vi "Begin.vi"(11 "Image Size":T1=enum."160x120") -> (0 "error out":errorcluster)   [LabVIEW 2013]
doc: "Called before other user functions, this VI is expected to open initial I/O refnums, load in file data, and do all program initialization. Notice that the <B>error out</B> terminal is simply used for data flow. Wiring it to other structures or subVIs ensures that this VI runs first."
uses:
  <vilib>/Rock Robotics/WPI/Camera/WPI_CameraImageSize.ctl
  <vilib>/Rock Robotics/WPI/Camera/WPI_CameraWhite Balance Values.ctl
  <vilib>/Rock Robotics/WPI/Camera/WPI_CameraExposure Values.ctl
  <vilib>/Rock Robotics/WPI/Camera/WPI_CameraFrameRate.ctl
  <vilib>/Rock Robotics/WPI/SafetyOutput/WPI_SafetyOutputConfigMenu.ctl
  <vilib>/Rock Robotics/WPI/DriverStation/WPI_DriverStationRobotMode2.ctl
  <vilib>/Rock Robotics/WPI/Joystick/WPI_JoystickDeviceEnum.ctl
  <vilib>/Rock Robotics/WPI/CAN/Jaguar/SubVIs/WPI_CANJaguar_ControlMode.ctl
  <vilib>/Rock Robotics/SystemInterfaces/DIO/FPGA_DIOPWMChannel.ctl
  <vilib>/Rock Robotics/SystemInterfaces/Typedef/FPGA_TypedefDigitalModule.ctl
  <vilib>/Rock Robotics/SystemInterfaces/DIO/FPGA_DIOChannel.ctl
  <vilib>/Rock Robotics/SystemInterfaces/AI/FPGA_AIChannel.ctl
  Robot Global Data.vi
  <vilib>/Rock Robotics/WPI/RobotDrive/WPI_RobotDriveOpen4MotorWithCANJaguar.vi
  <vilib>/Rock Robotics/WPI/MotorControl/WPI_MotorControlOpenCANJaguar.vi
  <vilib>/Rock Robotics/WPI/MotorControl/WPI_MotorControlOpen Victor.vi
  <vilib>/Rock Robotics/WPI/Relay/WPI_RelayDirection.ctl
  <vilib>/Rock Robotics/SystemInterfaces/DIO/FPGA_DIORelayChannel.ctl
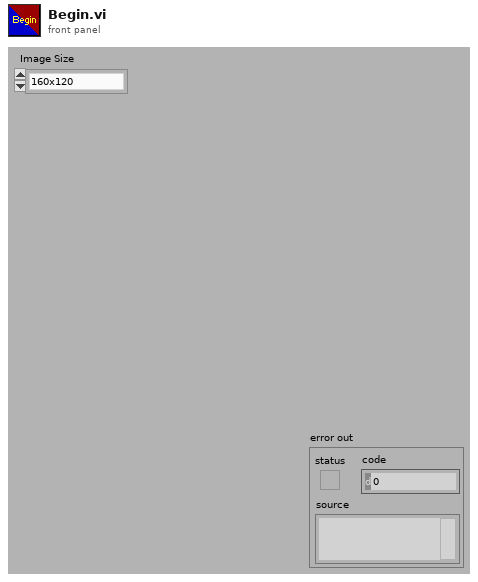
[diagram p1: front panel]
types:
  T1 = typedef "WPI_CameraImageSize.ctl" = enum16{"640x480", "320x240", "160x120"}
  T2 = typedef "FPGA_AIChannel.ctl" = enum8{"AI 1", "AI 2", "AI 3", "AI 4", "AI 5", "AI 6", "AI 7", "AI 8", "Invalid"}
  T3 = typedef "FPGA_DIOChannel.ctl" = enum8{"DIO 1", "DIO 2", "DIO 3", "DIO 4", "DIO 5", "DIO 6", "DIO 7", "DIO 8", "DIO 9", "DIO 10", "DIO 11", "DIO 12", "DIO 13", "DIO 14", "Invalid"}
  T4 = typedef "FPGA_DIOPWMChannel.ctl" = enum8{"PWM 1", "PWM 2", "PWM 3", "PWM 4", "PWM 5", "PWM 6", "PWM 7", "PWM 8", "PWM 9", "PWM 10", "Invalid"}
  T5 = typedef "FPGA_TypedefDigitalModule.ctl" = enum16{"Digital Module 1", "Digital Module 2"}
  T6 = typedef "WPI_CANJaguar_ControlMode.ctl" = enum8{"Percent VBus", "Current", "Speed", "Position", "Voltage"}
  T7 = typedef "WPI_JoystickDeviceEnum.ctl" = enum16{"USB 1", "USB 2", "USB 3", "USB 4", "Kinect 1", "Kinect 2"}
  T8 = typedef "WPI_DriverStationRobotMode2.ctl" = enum16{"Autonomous Disabled", "Autonomous Enabled", "Teleop Disabled", "Teleop Enabled", "Timeout", "Finish", "Test Disabled", "Test Enabled"}
  T9 = typedef "WPI_SafetyOutputConfigMenu.ctl" = enum16{"Enable", "Disable"}
  T10 = typedef "WPI_CameraFrameRate.ctl" = u32
  T11 = typedef "WPI_CameraExposure Values.ctl" = enum16{"Auto", "Flicker-free 50 Hz", "Flicker-free 60 Hz", "Hold current"}
  T12 = typedef "WPI_CameraWhite Balance Values.ctl" = enum16{"Auto", "Fixed indoor", "Fixed outdoor 1", "Fixed outdoor 2", "Fixed fluorescent 1", "Fixed fluorescent 2", "Hold current"}
  T13 = typedef "WPI_RelayDirection.ctl" = enum16{"Both directions", "Forward only", "Reverse only"}
  T14 = typedef "FPGA_DIORelayChannel.ctl" = enum8{"Relay 1", "Relay 2", "Relay 3", "Relay 4", "Relay 5", "Relay 6", "Relay 7", "Relay 8", "Invalid"}
  T15 = typedef "WPI_RelayDevRef.ctl" = cluster{"DevStatus":errorcluster, "Relay Channel":T14, "Digital Module":T5, "Relay Direction":T13}
  T16 = typedef "WPI_CameraDevRef.ctl" = cluster{"Camera Address":string, "CameraStatus":errorcluster, "Acquire Image Notifier":refnum<notifier>}
  T17 = typedef "WPI_RobotDriveDevRef.ctl" = cluster{"DevStatus":errorcluster, "Motors[]":T18[], "Square Inputs":bool, "Max Output":dbl, "Isochronous":bool}
  T18 = typedef "WPI_MotorControlDeviceRef.ctl" = cluster{"DeviceStatus":errorcluster, "Type":enum16{"PWM", "CAN"}, "PWM":cluster{"Digital Module":T5, "PWM Channel":T4, "DeadBand":T19}, "CAN":cluster{"Device Number":u8, "Control Mode":T6, "Semaphore":T20, "Max Vout":dbl}, "Invert":bool, "TransformRef":T21, "InvTransformRef":T21}
  T19 = typedef "WPI_PWMDeadband.ctl" = cluster{"Name":string, "maxPositivePwm":i32, "minPositivePwm":i32, "centerPwm":i32, "maxNegativePwm":i32, "minNegativePwm":i32, "angularRange":u16}
  T20 = typedef "Semaphore RefNum" = refnum<k1>
  T21 = typedef "WPI_PWMTransform_ConPane.ctl" = refnum<vi>
  T22 = typedef "WPI_ServoDeviceRef.ctl" = cluster{"DeviceStatus":errorcluster, "Digital Module":T5, "PWM Channel":T4, "DeadBand":T19}
  T23 = typedef "WPI_JoystickDevRef.ctl" = cluster{"Device":T7}
  T24 = typedef "WPI_AnalogChannelDevRef.ctl" = cluster{"DevStatus":errorcluster, "Analog Module":T25, "Analog Channel":T2}
  T25 = typedef "FPGA_TypedefAnalogModule.ctl" = enum16{"Analog Module 1", "Analog Module 2"}
  T26 = typedef "WPI_DigitalInputDevRef.ctl" = cluster{"DevStatus":errorcluster, "DIO Channel":T3, "Digital Module":T5}
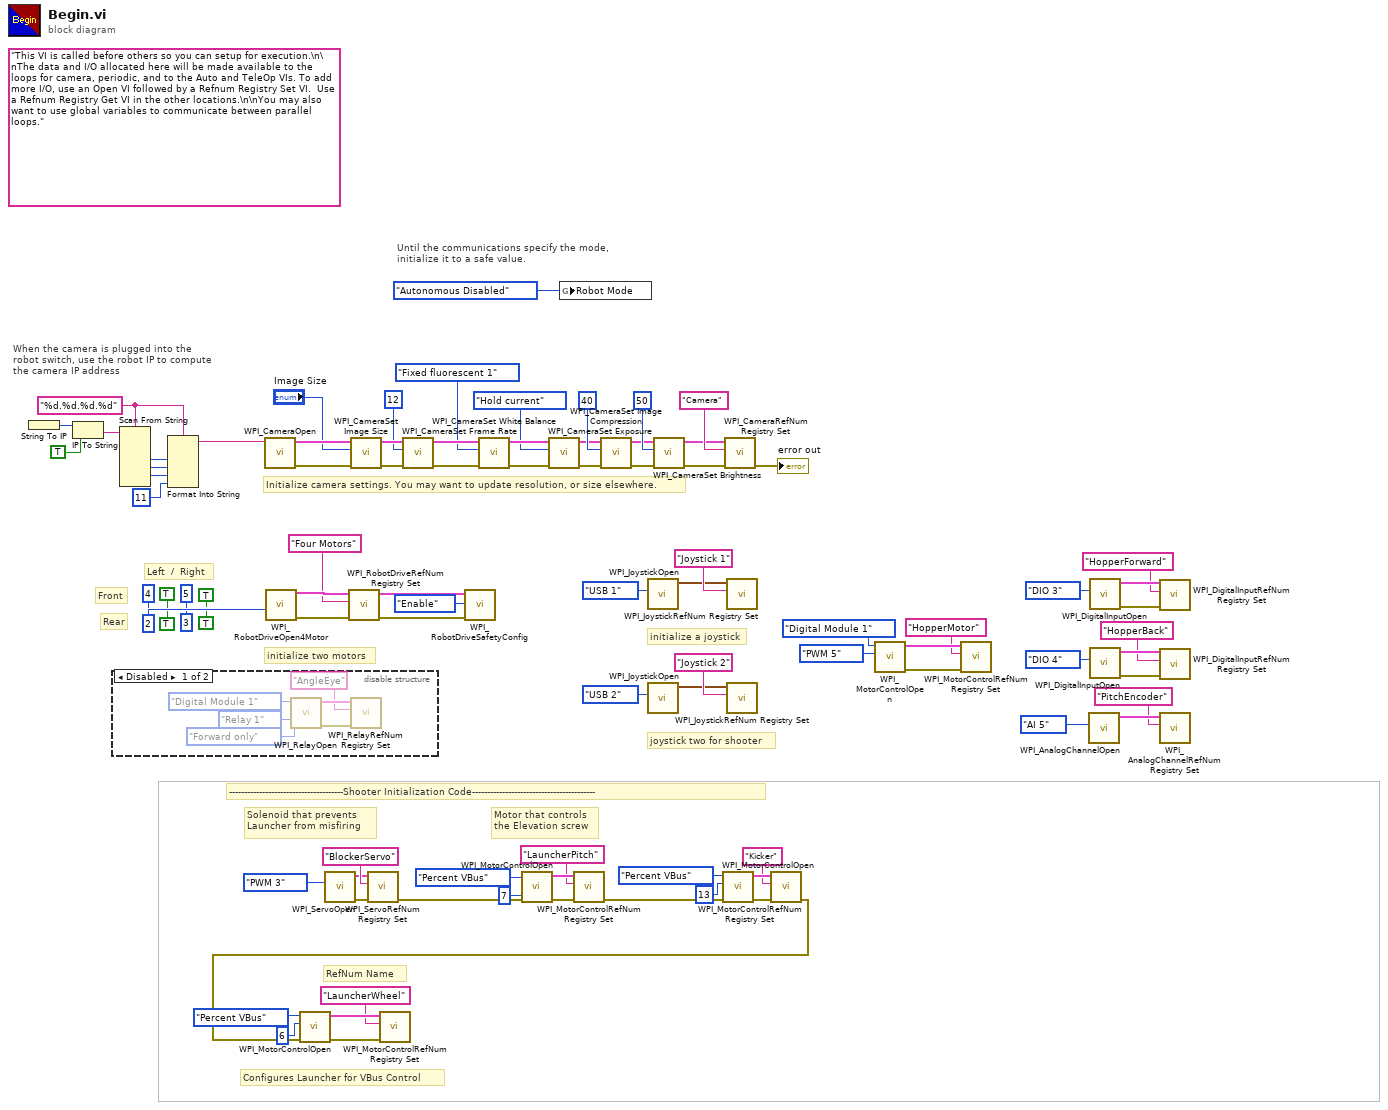
[diagram p0: block diagram]
diagram:
  w59 = "%d.%d.%d.%d" ("format string")
  (unwired) "This VI is called before others so you can setup for execution.\n\nThe data and I/O allocated here will be made available to the loops for camera, periodic, and to the Auto and TeleOp VIs. To add more I/O, use an Open VI followed by a Refnum Registry Set VI.  Use a Refnum Registry Get VI in the other locations.\n\nYou may also want to use global variables to communicate between parallel loops."
  # "Configures Launcher for VBus Control"
  # "RefNum Name"
  # "Motor that controls\nthe Elevation screw"
  # "Solenoid that prevents\nLauncher from misfiring"
  # "--------------------------------------Shooter Initialization Code-----------------------------------------"
  # "joystick two for shooter"
  # "Left  /  Right"
  # "Rear"
  # "Front"
  # "initialize a joystick"
  # "Until the communications specify the mode,\ninitialize it to a safe value."
  # "When the camera is plugged into the\nrobot switch, use the robot IP to compute\nthe camera IP address"
  # "initialize two motors"
  # "Initialize camera settings. You may want to update resolution, or size elsewhere."
  n1 = String To IP() -> (0:w66:u32)  [unwired: 1 in]
  n2 = IP To String(1:TRUE ("dot notation? (F)"), 2:w66) -> (0:w64:string)
  n3 = disable-structure shown="Disabled" {
    frame Disabled {
      n4 = call <vilib>:"WPI_RelayOpen.vi"("Relay Direction"=WPI_RelayDirection."Forward only", "Relay Channel"=FPGA_DIORelayChannel."Relay 1", "Digital Module (Module 1)"=FPGA_TypedefDigitalModule."Digital Module 1") -> ("error out"=w95:errorcluster, "RelayDevRef"=w96:T15)  [unwired: 7 in]
      n5 = call <vilib>:"WPI_RelayRefNum Registry Set.vi"("error in (no error)"=w95, "refnum name"="AngleEye", "RelayDevRef"=w96) -> ()  [unwired: 7 in, 2 out]
    }
    frame Enabled {
    }
  }
  n6 = Scan From String(format string=w59, input string=w64) -> (output 1=w63:i32, output 2=w62:i32, output 3=w61:i32)  [unwired: 7 in, 3 out]
  n7 = Format Into String(format string=w59, w63, w62, w61, 11 ("Compression")) -> (resulting string=w55:string)  [unwired: 2 in, 1 out]
  n8 = call <vilib>:"WPI_CameraOpen.vi"("Camera Address"=w55) -> ("error out"=w78:errorcluster, "CameraDevRef"=w79:T16)  [unwired: 1 in, 8 out]
  n9 = call-poly <vilib>:"WPI_RobotDriveOpen4Motor.vi"("Rear Left Motor"=u8 2, "Rear Left Motor Inverted"=TRUE, "Rear Right Motor Inverted"=TRUE, "Rear Right Motor"=u8 3, "Front Left Motor"=u8 4, "Front Right Motor"=u8 5, "Front Left Motor Inverted"=TRUE, "Front Right Motor Inverted"=TRUE) -> ("RobotDriveDevRef"=w89:T17, "error out"=w87:errorcluster)  [unwired: 6 in]
  n10 = call <vilib>:"WPI_ServoOpen.vi"("PWM Channel"=FPGA_DIOPWMChannel."PWM 3") -> ("error out"=w40:errorcluster, "ServoDeviceRef"=w19:T22)  [unwired: 9 in]
  n11 = call <vilib>:"WPI_RobotDriveRefNum Registry Set.vi"("error in (no error)"=w87, "refnum name"="Four Motors", "RobotDriveDevRef"=w89) -> ("error out"=w20:errorcluster, "RobotDriveDevRef"=w58:T17)  [unwired: 7 out]
  n12 = call <vilib>:"WPI_CameraSet Image Size.vi"("error in (no error)"=w78, "Image Size"="Image Size", "CameraDevRef"=w79) -> ("error out"=w77:errorcluster, "CameraDevRef Out"=w80:T16)  [unwired: 7 out]
  n13 = call <vilib>:"WPI_ServoRefNum Registry Set.vi"("error in (no error)"=w40, "refnum name"="BlockerServo", "ServoDeviceRef"=w19) -> ("error out"=w23:errorcluster)  [unwired: 7 in, 1 out]
  n14 = call <vilib>:"WPI_CameraSet Frame Rate.vi"("error in (no error)"=w77, "Frame Rate (fps)"=T10 12, "CameraDevRef"=w80) -> ("error out"=w76:errorcluster, "CameraDevRef Out"=w82:T16)  [unwired: 7 out]
  n15 = call <vilib>:"WPI_RobotDriveSafetyConfig.vi"("error in (no error)"=w20, "mode"=WPI_SafetyOutputConfigMenu."Enable", "RobotDriveDevRef"=w58) -> ()  [unwired: 7 in, 2 out]
  n16 = call <vilib>:"WPI_CameraSet White Balance.vi"("error in (no error)"=w76, "White Balance"=WPI_CameraWhite_Balance_Values."Fixed fluorescent 1", "CameraDevRef"=w82) -> ("error out"=w75:errorcluster, "CameraDevRef Out"=w81:T16)  [unwired: 7 out]
  n17 = call-poly <vilib>:"WPI_MotorControlOpen.vi"("error in (no error)"=w23, "Device Number"=u8 7, "Control Mode"=WPI_CANJaguar_ControlMode."Percent VBus") -> ("error out"=w35:errorcluster, "MotorControlDeviceRef"=w36:T18)  [unwired: 7 in]
  n18 = call <vilib>:"WPI_CameraSet Exposure.vi"("error in (no error)"=w75, "Exposure"=WPI_CameraExposure_Values."Hold current", "CameraDevRef"=w81) -> ("error out"=w74:errorcluster, "CameraDevRef Out"=w84:T16)  [unwired: 7 out]
  n19 = global write "Robot Global Data.vi" "Robot Mode"(WPI_DriverStationRobotMode2."Autonomous Disabled" ("Robot Mode")) -> ()
  n20 = call <vilib>:"WPI_MotorControlRefNum Registry Set.vi"("error in (no error)"=w35, "refnum name"="LauncherPitch", "MotorControlDevRef"=w36) -> ("error out"=w22:errorcluster)  [unwired: 7 in, 1 out]
  n21 = call <vilib>:"WPI_CameraSet Image Compression.vi"("error in (no error)"=w74, "Compression"=40, "CameraDevRef"=w84) -> ("error out"=w73:errorcluster, "CameraDevRef Out"=w83:T16)  [unwired: 7 out]
  n22 = call <vilib>:"WPI_JoystickOpen.vi"("JoystickDevice"=WPI_JoystickDeviceEnum."USB 1") -> ("JoystickDevRef"=w53:T23)  [unwired: 10 in]
  n23 = call <vilib>:"WPI_JoystickOpen.vi"("JoystickDevice"=WPI_JoystickDeviceEnum."USB 2") -> ("JoystickDevRef"=w42:T23)  [unwired: 10 in]
  n24 = call <vilib>:"WPI_CameraSet Brightness.vi"("error in (no error)"=w73, "Brightness"=50, "CameraDevRef"=w83) -> ("error out"=w71:errorcluster, "CameraDevRef Out"=w72:T16)  [unwired: 7 out]
  n25 = call-poly <vilib>:"WPI_MotorControlOpen.vi"("error in (no error)"=w22, "Device Number"=u8 13, "Control Mode"=WPI_CANJaguar_ControlMode."Percent VBus") -> ("error out"=w27:errorcluster, "MotorControlDeviceRef"=w28:T18)  [unwired: 7 in]
  n26 = call <vilib>:"WPI_CameraRefNum Registry Set.vi"("error in (no error)"=w71, "refnum name"="Camera", "CameraDevRef"=w72) -> ("error out"=→"error out":errorcluster)  [unwired: 8 out]
  n27 = call <vilib>:"WPI_JoystickRefNum Registry Set.vi"("refnum name"="Joystick 1", "JoystickDevRef"=w53) -> ()  [unwired: 8 in, 2 out]
  n28 = call <vilib>:"WPI_JoystickRefNum Registry Set.vi"("refnum name"="Joystick 2", "JoystickDevRef"=w42) -> ()  [unwired: 8 in, 2 out]
  n29 = call <vilib>:"WPI_MotorControlRefNum Registry Set.vi"("error in (no error)"=w27, "refnum name"="Kicker", "MotorControlDevRef"=w28) -> ("error out"=w21:errorcluster)  [unwired: 7 in, 1 out]
  n30 = call-poly <vilib>:"WPI_MotorControlOpen.vi"("error in (no error)"=w21, "Device Number"=u8 6, "Control Mode"=WPI_CANJaguar_ControlMode."Percent VBus") -> ("error out"=w31:errorcluster, "MotorControlDeviceRef"=w30:T18)  [unwired: 7 in]
  n31 = call <vilib>:"WPI_MotorControlRefNum Registry Set.vi"("error in (no error)"=w31, "refnum name"="LauncherWheel", "MotorControlDevRef"=w30) -> ()  [unwired: 7 in, 2 out]
  n32 = call-poly <vilib>:"WPI_MotorControlOpen.vi"("PWM Channel"=FPGA_DIOPWMChannel."PWM 5", "Digital Module (Module 1)"=FPGA_TypedefDigitalModule."Digital Module 1") -> ("error out"=w14:errorcluster, "MotorControlDeviceRef"=w17:T18)  [unwired: 8 in]
  n33 = call <vilib>:"WPI_MotorControlRefNum Registry Set.vi"("error in (no error)"=w14, "refnum name"="HopperMotor", "MotorControlDevRef"=w17) -> ()  [unwired: 7 in, 2 out]
  n34 = call <vilib>:"WPI_AnalogChannelOpen.vi"("Analog Channel"=FPGA_AIChannel."AI 5") -> ("AIDeviceRef"=w3:T24)  [unwired: 9 in, 1 out]
  n35 = call <vilib>:"WPI_DigitalInputOpen.vi"("DIO Channel"=FPGA_DIOChannel."DIO 3") -> ("error out"=w10:errorcluster, "DigitalInputDevRef"=w12:T26)  [unwired: 9 in]
  n36 = call <vilib>:"WPI_DigitalInputOpen.vi"("DIO Channel"=FPGA_DIOChannel."DIO 4") -> ("error out"=w7:errorcluster, "DigitalInputDevRef"=w8:T26)  [unwired: 9 in]
  n37 = call <vilib>:"WPI_DigitalInputRefNum Registry Set.vi"("error in (no error)"=w10, "refnum name"="HopperForward", "DigitalInputDevRef"=w12) -> ()  [unwired: 7 in, 2 out]
  n38 = call <vilib>:"WPI_DigitalInputRefNum Registry Set.vi"("error in (no error)"=w7, "refnum name"="HopperBack", "DigitalInputDevRef"=w8) -> ()  [unwired: 7 in, 2 out]
  n39 = call <vilib>:"WPI_AnalogChannelRefNum Registry Set.vi"("refnum name"="PitchEncoder", "AIDeviceRef"=w3) -> ()  [unwired: 8 in, 2 out]
